vi "Handle Events.vi"(8 "error in (no error)":errorcluster, 11 "TreeControlEventHandler":refnum<class "TreeControlEventHandler.lvclass">) -> ()   [LabVIEW 2019, in "ActorEvents.lvlib" / "TreeControlEventHandler.lvclass"]
uses:
  <vilib>/gpm_packages/@cs/mva-viewable/Source/ActorEvents/EventHandler/TreeControlEventHandler/TreeControlEventHandler.lvclass
  C:/Program Files/National Instruments/LabVIEW 2019/vi.lib/gpm_packages/@cs/mva-viewable/Source/ActorEvents/IEventHandler/IEventHandler.lvclass
  <vilib>/gpm_packages/@cs/mva-viewable/Source/ActorEvents/EventHandler/TreeControlEventHandler/TreeControlEventHandler.lvclass/TreeControlEventHandler.ctl
  <vilib>/gpm_packages/@cs/mva-viewable/Source/ActorEvents/IEventHandler/IEventHandler.lvclass/IEventHandler.ctl
  <vilib>/ActorFramework/Message Enqueuer/Message Enqueuer.lvclass/Message Enqueuer.ctl
  <vilib>/gpm_packages/@cs/mva-viewable/Source/ActorEvents/IEventAggregator Messages/EventDataMessage/EventDataMessage.lvclass/EventDataMessage.ctl
  <vilib>/gpm_packages/@cs/mva-viewable/Source/ActorEvents/IEventAggregator Messages/ControlDragSourceUpdateMsg/ControlDragSourceUpdateMsg.lvclass/ControlDragSourceUpdateMsg.ctl
  <vilib>/gpm_packages/@cs/mva-viewable/Source/ActorEvents/IEventAggregator Messages/ControlDragStartingMsg/ControlDragStartingMsg.lvclass/ControlDragStartingMsg.ctl
  <vilib>/gpm_packages/@cs/mva-viewable/Source/ActorEvents/IEventAggregator Messages/ControlMouseDownMsg/ControlMouseDownMsg.lvclass/ControlMouseDownMsg.ctl
  <vilib>/gpm_packages/@cs/mva-viewable/Source/ActorEvents/IEventAggregator Messages/ControlKeyDownMsg/ControlKeyDownMsg.lvclass/ControlKeyDownMsg.ctl
  <vilib>/event_ctls.llb/lveventtype.ctl
  <vilib>/gpm_packages/@cs/mva-viewable/Source/ActorEvents/IEventAggregator Messages/TreeEditCellMsg/TreeEditCellMsg.lvclass/TreeEditCellMsg.ctl
  <vilib>/gpm_packages/@cs/mva-viewable/Source/ActorEvents/IEventAggregator Messages/EventDataMessage/Read Discarded.vi
  <vilib>/gpm_packages/@cs/mva-viewable/Source/ActorEvents/IEventAggregator Messages/ControlDragSourceUpdateMsg/Accessors/Read Cursor.vi
  <vilib>/gpm_packages/@cs/mva-viewable/Source/ActorEvents/IEventAggregator Messages/ControlDragStartingMsg/Accessors/Read Data.vi
  <vilib>/gpm_packages/@cs/mva-viewable/Source/ActorEvents/IEventAggregator Messages/ControlDragStartingMsg/Accessors/Read Drag Mode.vi
  <vilib>/gpm_packages/@cs/mva-viewable/Source/ActorEvents/IEventAggregator Messages/ControlMouseDownMsg/Accessors/Read Button.vi
  <vilib>/gpm_packages/@cs/mva-viewable/Source/ActorEvents/IEventAggregator Messages/ControlMouseDownMsg/Accessors/Read Mods.vi
  <vilib>/gpm_packages/@cs/mva-viewable/Source/ActorEvents/IEventAggregator Messages/ControlMouseDownMsg/Accessors/Read PlatMods.vi
  <vilib>/gpm_packages/@cs/mva-viewable/Source/ActorEvents/IEventAggregator Messages/ControlKeyDownMsg/Accessors/Read Char.vi
  <vilib>/gpm_packages/@cs/mva-viewable/Source/ActorEvents/IEventAggregator Messages/ControlKeyDownMsg/Accessors/Read VKey.vi
  <vilib>/gpm_packages/@cs/mva-viewable/Source/ActorEvents/IEventAggregator Messages/ControlKeyDownMsg/Accessors/Read Mods.vi
  <vilib>/gpm_packages/@cs/mva-viewable/Source/ActorEvents/IEventAggregator Messages/ControlKeyDownMsg/Accessors/Read PlatMods.vi
  <vilib>/gpm_packages/@cs/mva-viewable/Source/ActorEvents/IEventAggregator Messages/ControlKeyDownMsg/Accessors/Read FocusObj.vi
  <vilib>/gpm_packages/@cs/mva-viewable/Source/ActorEvents/IEventAggregator Messages/TreeEditCellMsg/Accessors/Read String.vi
  <vilib>/gpm_packages/@cs/mva-viewable/Source/ActorEvents/IEventHandler/Accessors/Read Timeout [ms].vi
  <vilib>/gpm_packages/@cs/mva-viewable/Source/ActorEvents/IEventHandler/Accessors/Read Event Filter.vi
  <vilib>/gpm_packages/@cs/mva-viewable/Source/ActorEvents/IEventHandler/Accessors/Read EventAggregator Enqueuer.vi
  <vilib>/gpm_packages/@cs/mva-viewable/Source/ActorEvents/IEventHandler/Accessors/Read Timeout Message.vi
  <vilib>/gpm_packages/@cs/mva-viewable/Source/ActorEvents/IEventHandler/Accessors/Read Timeout Message Priority.vi
  <vilib>/gpm_packages/@cs/mva-viewable/Source/ActorEvents/IEventAggregator Messages/ControlDropMsg/ControlDropMsg.lvclass
  C:/Program Files/National Instruments/LabVIEW 2019/vi.lib/gpm_packages/@cs/mva-viewable/Source/ActorEvents/IEventAggregator Messages/EventDataMessage/EventDataMessage.lvclass
  <vilib>/gpm_packages/@cs/mva-viewable/Source/ActorEvents/IEventAggregator Messages/ControlDragOverMsg/ControlDragOverMsg.lvclass
  <vilib>/gpm_packages/@cs/mva-viewable/Source/ActorEvents/IEventAggregator Messages/ControlDragSourceUpdateMsg/ControlDragSourceUpdateMsg.lvclass
  <vilib>/gpm_packages/@cs/mva-viewable/Source/ActorEvents/IEventAggregator Messages/ControlDragStartingMsg/ControlDragStartingMsg.lvclass
  <vilib>/gpm_packages/@cs/mva-viewable/Source/ActorEvents/IEventAggregator Messages/ControlMouseDownMsg/ControlMouseDownMsg.lvclass
  <vilib>/gpm_packages/@cs/mva-viewable/Source/ActorEvents/IEventAggregator Messages/ControlKeyDownMsg/ControlKeyDownMsg.lvclass
  <vilib>/gpm_packages/@cs/mva-viewable/Source/ActorEvents/IEventAggregator Messages/TreeItemOpenMsg/TreeItemOpenMsg.lvclass
  <vilib>/gpm_packages/@cs/mva-viewable/Source/ActorEvents/IEventAggregator Messages/TreeItemCloseMsg/TreeItemCloseMsg.lvclass
  <vilib>/gpm_packages/@cs/mva-viewable/Source/ActorEvents/IEventAggregator Messages/ShortcutMenuActivationMsg/ShortcutMenuActivationMsg.lvclass
  <vilib>/gpm_packages/@cs/mva-viewable/Source/ActorEvents/IEventAggregator Messages/ShortcutMenuSelectionMsg/ShortcutMenuSelectionMsg.lvclass
  <vilib>/gpm_packages/@cs/mva-viewable/Source/ActorEvents/IEventAggregator Messages/TreeEditCellMsg/TreeEditCellMsg.lvclass
  <vilib>/ActorFramework/Message Priority Queue/Priority Enqueue.vi
  <vilib>/gpm_packages/@cs/mva-viewable/Source/ActorEvents/IEventFilter/IEventFilter.lvclass
  <vilib>/ActorFramework/Message Enqueuer/Message Enqueuer.lvclass
  <vilib>/ActorFramework/Message/Message.lvclass
  <vilib>/gpm_packages/@cs/mva-viewable/Source/ActorEvents/IEventAggregator Messages/ValueChangeMsg/ValueChangeMsg.lvclass
  <vilib>/gpm_packages/@cs/mva-viewable/Source/ActorEvents/IEventAggregator Messages/ControlMouseUpMsg/ControlMouseUpMsg.lvclass
  <vilib>/gpm_packages/@cs/mva-viewable/Source/ActorEvents/IEventAggregator Messages/TreeDoubleClickMsg/TreeDoubleClickMsg.lvclass
  <vilib>/gpm_packages/@cs/mva-viewable/Source/ActorEvents/IEventAggregator Messages/ControlMouseEnterMsg/ControlMouseEnterMsg.lvclass
  <vilib>/gpm_packages/@cs/mva-viewable/Source/ActorEvents/IEventAggregator Messages/ControlMouseLeaveMsg/ControlMouseLeaveMsg.lvclass
  <vilib>/gpm_packages/@cs/mva-viewable/Source/ActorEvents/IEventAggregator Messages/ControlKeyUpMsg/ControlKeyUpMsg.lvclass
  <vilib>/gpm_packages/@cs/mva-viewable/Source/ActorEvents/IEventAggregator Messages/ControlDragEndedMsg/ControlDragEndedMsg.lvclass
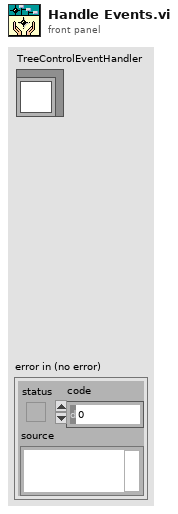
[diagram p1: front panel]
types:
  T1 = typedef "ActorEvents.lvlib/IEventFilter.lvclass/EventFilter Reference.ctl" = refnum<data-value>
  T2 = typedef "Actor Framework.lvlib/Message Enqueuer.lvclass/Message Priority.ctl" = enum16{"Low", "Normal", "High"}
  T3 = typedef "lveventtype.ctl" = enum32{"Null", "Timeout", "Annotation Menu Selection", "Annotation Menu Selection?", "App Instance Close", "App Instance Close?", "Autoscale Range Change", "Bookmark Info Change", "Cell Edit", "Cell Edit?", "Cursor Grab", "Cursor Grab?", "Cursor Menu Selection", "Cursor Menu Selection?", "Cursor Move", "Cursor Release", "Data Change", "Direction Change", "Display State Change", "Drag Ended", "Drag Enter", "Drag Leave", "Drag Over", "Drag Source Update", "Drag Starting", "Drag Starting?", "Drop", "Exec State Change", "Key Down", "Key Down?", "Key Repeat", "Key Repeat?", "Key Up", "Listbox Double Click", "Menu Activation?", "Menu Selection (App)", "Menu Selection? (App)", "Menu Selection (User)", "Mouse Down", "Mouse Down?", "Mouse Enter", "Mouse Leave", "Mouse Move", "Mouse Up", "Mouse Wheel", "NI Security User Change (App)", "Pane Size", "Panel Close", "Panel Close?", "Panel Resize", "Plot Attribute Change", "Scale Range Change", "Shortcut Menu Activation?", "Shortcut Menu Selection (App)", "Shortcut Menu Selection? (App)", "Shortcut Menu Selection (User)", "Tree Double Click", "Tree Drag", "Tree Drag?", "Tree Drop", "Tree Drop?", "Tree Item Close", "Tree Item Close?", "Tree Item Open", "Tree Item Open?", "User Event", "Value Change"}
  T4 = typedef "LVPoint32TypeDef.ctl" = cluster{"Horizontal":i32, "Vertical":i32}
  T5 = cluster{"Shift":bool, "Ctrl":bool, "Alt":bool, "Cmd":bool, "Opt":bool}
  T6 = cluster{"data name":string, "drag data":variant}[]
  T7 = typedef "eventvkey.ctl" = enum16{"ASCII", "Enter", "Return", "Shift", "Ctrl", "Alt", "Cmd", "Opt", "Caps", "NumLock", "Clear", "Break", "Up", "Down", "Left", "Right", "Insert", "Delete", "Home", "End", "PageUp", "PageDown", "Escape", "Help", "Pause", "ScrollLock", "F1", "F2", "F3", "F4", "F5", "F6", "F7", "F8", "F9", "F10", "F11", "F12", "F13", "F14", "F15", "F16", "F17", "F18", "F19", "F20", "F21", "F22", "F23", "F24", "Play", "VolumeUp", "VolumeDown", "Mute", "Two Byte Char"}
  T8 = enum16{"Text", "Background", "Item Symbol", "Open/Close Symbol", "Hierarchy Lines", "Right Border", "Bottom Border", "Bottom Right Corner", "Unknown Part"}
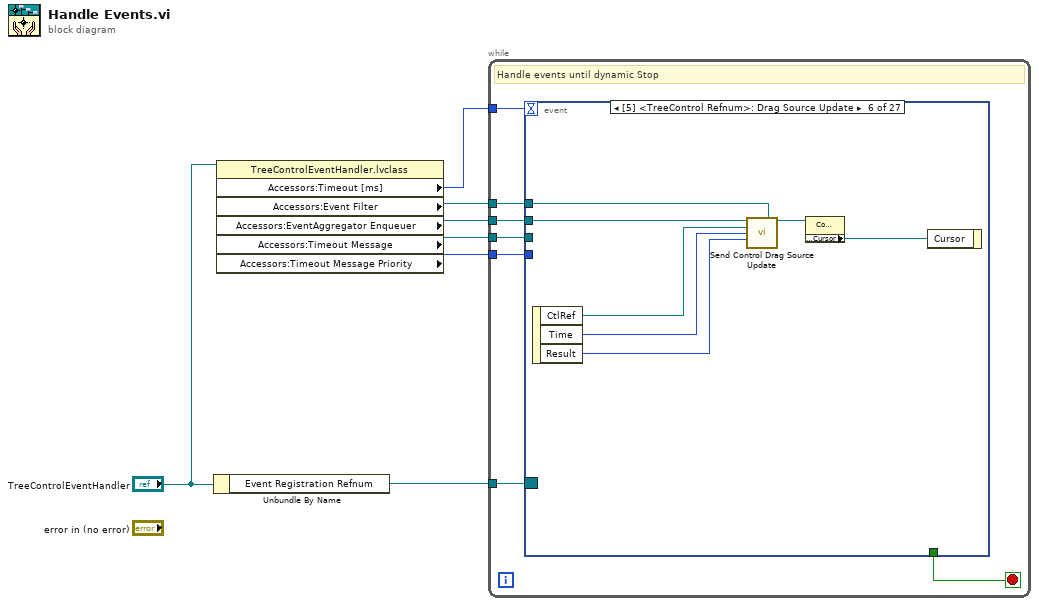
[diagram p0: block diagram]
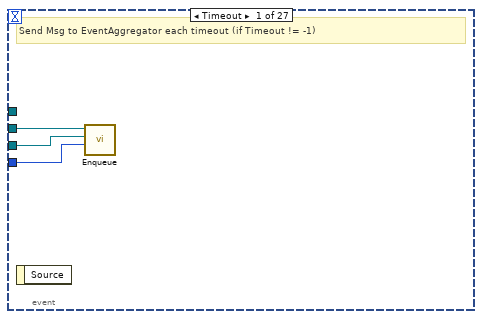
[diagram p2: hidden frame]
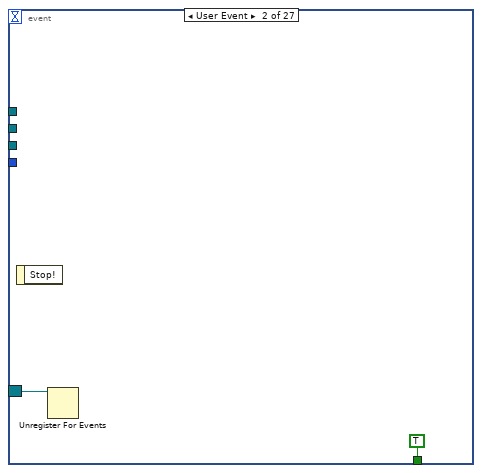
[diagram p3: hidden frame]
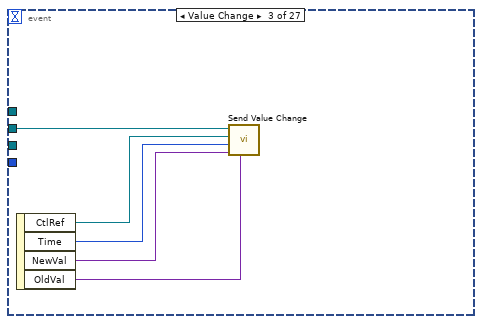
[diagram p4: hidden frame]
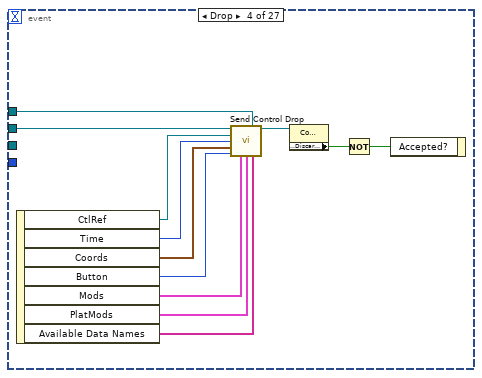
[diagram p5: hidden frame]
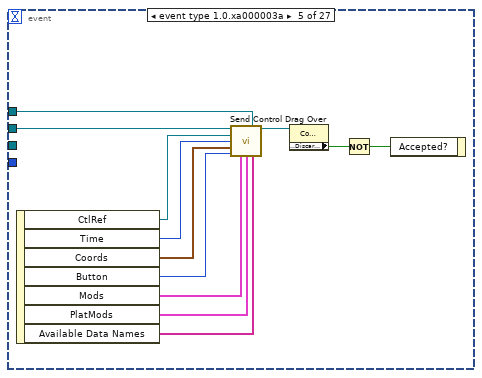
[diagram p6: hidden frame]
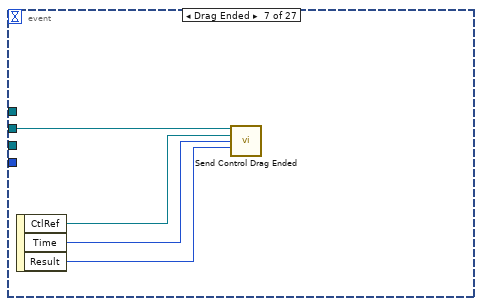
[diagram p7: hidden frame]
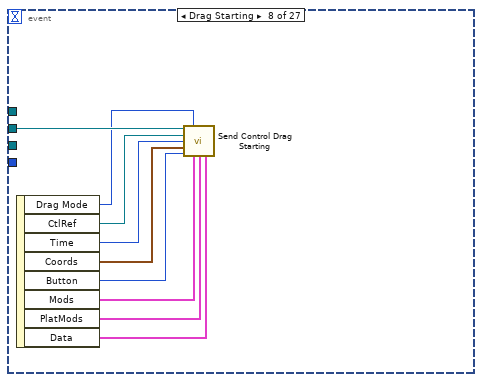
[diagram p8: hidden frame]
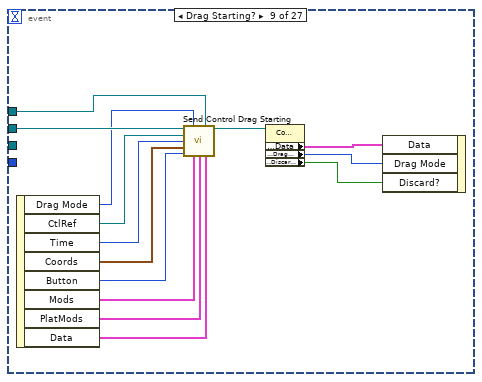
[diagram p9: hidden frame]
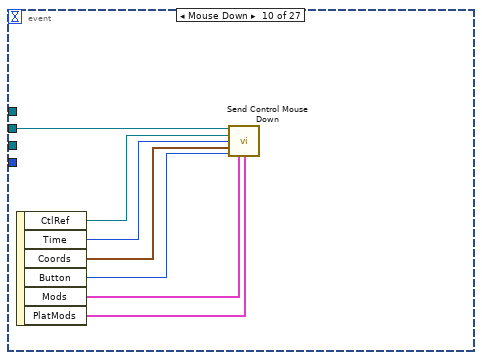
[diagram p10: hidden frame]
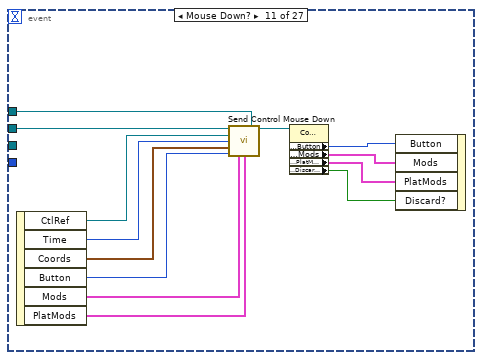
[diagram p11: hidden frame]
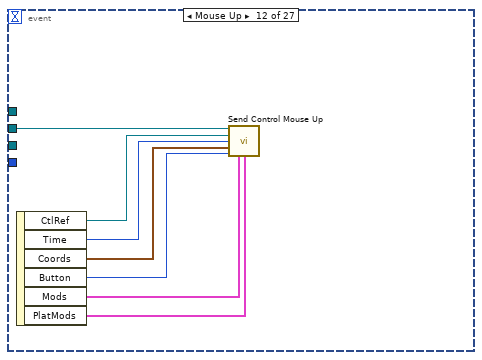
[diagram p12: hidden frame]
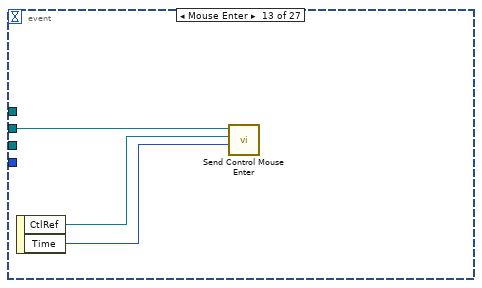
[diagram p13: hidden frame]
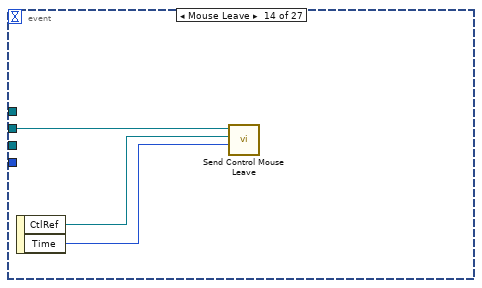
[diagram p14: hidden frame]
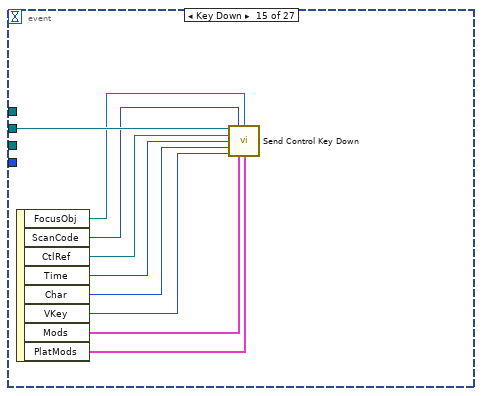
[diagram p15: hidden frame]
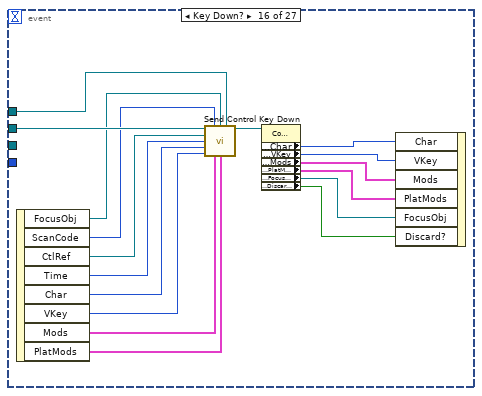
[diagram p16: hidden frame]
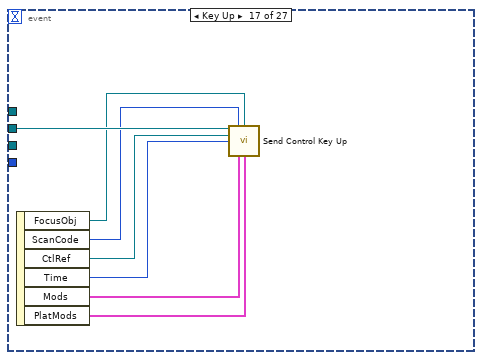
[diagram p17: hidden frame]
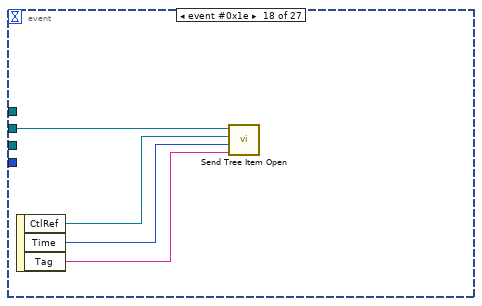
[diagram p18: hidden frame]
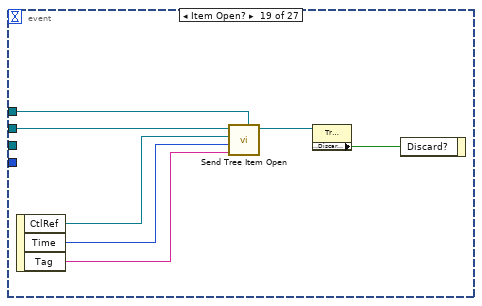
[diagram p19: hidden frame]
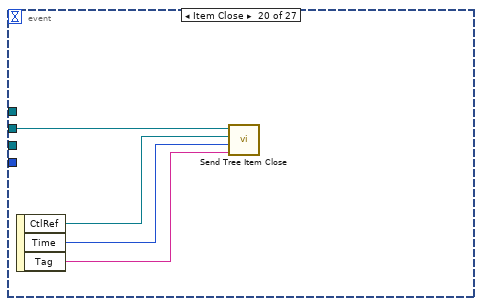
[diagram p20: hidden frame]
diagram:
  n1 = Unbundle By Name("TreeControlEventHandler") -> ("Event Registration Refnum"=w7:refnum<event-registration>)
  n2 = property class="TreeControlEventHandler.lvclass"(reference="TreeControlEventHandler") -> ("Accessors:Timeout [ms]"=w5:i32, "Accessors:Event Filter"=w1:T1, "Accessors:EventAggregator Enqueuer"=w4:refnum<class "Message Enqueuer.lvclass">, "Accessors:Timeout Message"=w3:refnum<class "Message.lvclass">, "Accessors:Timeout Message Priority"=w2:T2)  [unwired: 1 in, 2 out]
  n3 = while {
    tunnel: w7 -> [w14]
    tunnel: w4 -> [w13]
    tunnel: w3 -> [w12]
    tunnel: w5 -> [w11]
    tunnel: w2 -> [w9]
    tunnel: w1 -> [w8]
    stop <- w10 stop-if-true
    # "Handle events until dynamic Stop"
    n4 = event shown="[5] <TreeControl Refnum>: Drag Source Update" {
      selector: w14 -> [_ w19 _ _ _ _ _ _ _ _ _ _ _ _ _ _ _ _ _ _ _ _ _ _ _ _ _]
      dyn-events: _ -> [_ _ _ _ _ _ _ _ _ _ _ _ _ _ _ _ _ _ _ _ _ _ _ _ _ _ _]
      timeout: w11 -> [_ _ _ _ _ _ _ _ _ _ _ _ _ _ _ _ _ _ _ _ _ _ _ _ _ _ _]
      tunnel: [_ TRUE ("Stop!") _ _ _ _ _ _ _ _ _ _ _ _ _ _ _ _ _ _ _ _ _ _ _ _ _] -> w10
      tunnel: w13 -> [w17 _ w24 w36 w48 w55 w59 w68 w82 w89 w102 w109 w112 w115 w124 w141 w148 w152 w159 w163 w170 w179 w188 w198 w209 w215 w225]
      tunnel: w12 -> [w16 _ _ _ _ _ _ _ _ _ _ _ _ _ _ _ _ _ _ _ _ _ _ _ _ _ _]
      tunnel: w9 -> [w15 _ _ _ _ _ _ _ _ _ _ _ _ _ _ _ _ _ _ _ _ _ _ _ _ _ _]
      tunnel: w8 -> [_ _ _ w28 w41 w52 _ _ w73 _ w95 _ _ _ _ w132 _ _ w155 _ w166 _ w182 _ w202 _ w219]
      event Timeout {
        # "Send Msg to EventAggregator each timeout (if Timeout != -1)"
        n5 = event-data() -> ()  [unwired: 1 in, 1 out]
        n6 = call <vilib>:"Enqueue.vi"("Message Priority (Normal)"=w15, "Message"=w16, "Message Enqueuer in"=w17) -> ()  [unwired: 7 in, 2 out]
      }
      event User Event {
        n7 = event-data() -> ()  [unwired: 1 in, 1 out]
        n8 = Unregister For Events(event registration refnum=w19) -> ()  [unwired: 1 in, 1 out]
      }
      event Value Change {
        n9 = event-data() -> ("CtlRef"=w21:refnum<vi>, "Time"=w23:u32, "NewVal"=w22:variant, "OldVal"=w20:variant)  [unwired: 1 in]
        n10 = call <vilib>:"Send Value Change.vi"("Old Value"=w20, "New Value"=w22, "Time"=w23, "Ctl Refnum"=w21, "Message Enqueuer in"=w24) -> ()  [unwired: 6 in, 1 out]
      }
      event Drop {
        n11 = event-data() -> ("CtlRef"=w35:refnum<vi>, "Time"=w34:u32, "Coords"=w33:T4, "Button"=w32:u16, "Mods"=w31:cluster{"Double Click":bool, "Menu Key":bool}, "PlatMods"=w30:T5, "Available Data Names"=w29:string[])  [unwired: 1 in]
        n12 = call <vilib>:"Send Control Drop.vi"("Message Enqueuer in"=w36, "EventFilter Reference"=w28, "CtlRef"=w35, "Time"=w34, "Coords"=w33, "Button"=w32, "Mods"=w31, "PlatMods"=w30, "Available Data Names"=w29) -> ("Filtered EventDataMessage"=w27:refnum<class "ControlDropMsg.lvclass">)  [unwired: 5 in, 1 out]
        n13 = property class="ControlDropMsg.lvclass"(reference=w27) -> ("Accessors:Discarded?"=w26:bool)  [unwired: 1 in, 2 out]
        n14 = Not(x=w26) -> (.not. x?=w25:bool)
        n15 = event-data("Accepted?"=w25) -> ()  [unwired: 1 in, 1 out]
      }
      event event type 1.0.xa000003a {
        n16 = event-data() -> ("CtlRef"=w47:refnum<vi>, "Time"=w46:u32, "Coords"=w45:T4, "Button"=w44:u16, "Mods"=w43:cluster{"Double Click":bool, "Menu Key":bool}, "PlatMods"=w42:T5, "Available Data Names"=w37:string[])  [unwired: 1 in]
        n17 = call <vilib>:"Send Control Drag Over.vi"("Message Enqueuer in"=w48, "EventFilter Reference"=w41, "CtlRef"=w47, "Time"=w46, "Coords"=w45, "Button"=w44, "Mods"=w43, "PlatMods"=w42, "Available Data Names"=w37) -> ("Filtered EventDataMessage"=w40:refnum<class "ControlDragOverMsg.lvclass">)  [unwired: 5 in, 1 out]
        n18 = property class="ControlDragOverMsg.lvclass"(reference=w40) -> ("Accessors:Discarded?"=w39:bool)  [unwired: 1 in, 2 out]
        n19 = Not(x=w39) -> (.not. x?=w38:bool)
        n20 = event-data("Accepted?"=w38) -> ()  [unwired: 1 in, 1 out]
      }
      event Drag Source Update {
        n21 = event-data() -> ("CtlRef"=w54:refnum<vi>, "Time"=w53:u32, "Result"=w49:enum16{"Drop Cancel", "Drop Move", "Drop Copy"})  [unwired: 1 in]
        n22 = call <vilib>:"Send Control Drag Source Update.vi"("Message Enqueuer in"=w55, "EventFilter Reference"=w52, "CtlRef"=w54, "Time"=w53, "Result"=w49) -> ("Filtered EventDataMessage"=w51:refnum<class "ControlDragSourceUpdateMsg.lvclass">)  [unwired: 9 in, 1 out]
        n23 = property class="ControlDragSourceUpdateMsg.lvcl"(reference=w51) -> ("Accessors:Cursor"=w50:refnum<k1>)  [unwired: 1 in, 2 out]
        n24 = event-data("Cursor"=w50) -> ()  [unwired: 1 in, 1 out]
      }
      event Drag Ended {
        n25 = event-data() -> ("CtlRef"=w58:refnum<vi>, "Time"=w57:u32, "Result"=w56:enum16{"Drop Cancel", "Drop Move", "Drop Copy"})  [unwired: 1 in]
        n26 = call <vilib>:"Send Control Drag Ended.vi"("Message Enqueuer in"=w59, "CtlRef"=w58, "Time"=w57, "Result"=w56) -> ()  [unwired: 10 in, 2 out]
      }
      event Drag Starting {
        n27 = event-data() -> ("Drag Mode"=w67:enum32{"copy or move", "copy only", "move only"}, "CtlRef"=w66:refnum<vi>, "Time"=w65:u32, "Coords"=w64:T4, "Button"=w63:u16, "Mods"=w62:cluster{"Double Click":bool, "Menu Key":bool}, "PlatMods"=w61:T5, "Data"=w60:T6)  [unwired: 1 in]
        n28 = call <vilib>:"Send Control Drag Starting.vi"("Message Enqueuer in"=w68, "Drag Mode"=w67, "CtlRef"=w66, "Time"=w65, "Coords"=w64, "Button"=w63, "Mods"=w62, "PlatMods"=w61, "Data"=w60) -> ()  [unwired: 5 in, 2 out]
      }
      event Drag Starting? {
        n29 = event-data() -> ("Drag Mode"=w81:enum32{"copy or move", "copy only", "move only"}, "CtlRef"=w80:refnum<vi>, "Time"=w79:u32, "Coords"=w78:T4, "Button"=w77:u16, "Mods"=w76:cluster{"Double Click":bool, "Menu Key":bool}, "PlatMods"=w75:T5, "Data"=w74:T6)  [unwired: 1 in]
        n30 = call <vilib>:"Send Control Drag Starting.vi"("Message Enqueuer in"=w82, "Drag Mode"=w81, "EventFilter Reference"=w73, "CtlRef"=w80, "Time"=w79, "Coords"=w78, "Button"=w77, "Mods"=w76, "PlatMods"=w75, "Data"=w74) -> ("Filtered EventDataMessage"=w72:refnum<class "ControlDragStartingMsg.lvclass">)  [unwired: 4 in, 1 out]
        n31 = property class="ControlDragStartingMsg.lvclass"(reference=w72) -> ("Accessors:Data"=w71:T6, "Accessors:Drag Mode"=w70:enum32{"copy or move", "copy only", "move only"}, "Accessors:Discarded?"=w69:bool)  [unwired: 1 in, 2 out]
        n32 = event-data("Data"=w71, "Drag Mode"=w70, "Discard?"=w69) -> ()  [unwired: 1 in, 1 out]
      }
      event Mouse Down {
        n33 = event-data() -> ("CtlRef"=w88:refnum<vi>, "Time"=w87:u32, "Coords"=w86:T4, "Button"=w85:u16, "Mods"=w84:cluster{"Double Click":bool, "Menu Key":bool}, "PlatMods"=w83:T5)  [unwired: 1 in]
        n34 = call <vilib>:"Send Control Mouse Down.vi"("Message Enqueuer in"=w89, "Ctl Refnum"=w88, "Time"=w87, "Coords"=w86, "Button"=w85, "Mods"=w84, "PlatMods"=w83) -> ()  [unwired: 7 in, 2 out]
      }
      event Mouse Down? {
        n35 = event-data() -> ("CtlRef"=w101:refnum<vi>, "Time"=w100:u32, "Coords"=w99:T4, "Button"=w98:u16, "Mods"=w97:cluster{"Double Click":bool, "Menu Key":bool}, "PlatMods"=w96:T5)  [unwired: 1 in]
        n36 = call <vilib>:"Send Control Mouse Down.vi"("Message Enqueuer in"=w102, "EventFilter Reference"=w95, "Ctl Refnum"=w101, "Time"=w100, "Coords"=w99, "Button"=w98, "Mods"=w97, "PlatMods"=w96) -> ("Filtered EventDataMessage"=w94:refnum<class "ControlMouseDownMsg.lvclass">)  [unwired: 6 in, 1 out]
        n37 = property class="ControlMouseDownMsg.lvclass"(reference=w94) -> ("Accessors:Button"=w93:u16, "Accessors:Mods"=w92:cluster{"Double Click":bool, "Menu Key":bool}, "Accessors:PlatMods"=w91:T5, "Accessors:Discarded?"=w90:bool)  [unwired: 1 in, 2 out]
        n38 = event-data("Button"=w93, "Mods"=w92, "PlatMods"=w91, "Discard?"=w90) -> ()  [unwired: 1 in, 1 out]
      }
      event Mouse Up {
        n39 = event-data() -> ("CtlRef"=w108:refnum<vi>, "Time"=w107:u32, "Coords"=w106:T4, "Button"=w105:u16, "Mods"=w104:cluster{"Double Click":bool, "Menu Key":bool}, "PlatMods"=w103:T5)  [unwired: 1 in]
        n40 = call <vilib>:"Send Control Mouse Up.vi"("Message Enqueuer in"=w109, "Ctl Refnum"=w108, "Time"=w107, "Coords"=w106, "Button"=w105, "Mods"=w104, "PlatMods"=w103) -> ()  [unwired: 8 in, 1 out]
      }
      event Mouse Enter {
        n41 = event-data() -> ("CtlRef"=w111:refnum<vi>, "Time"=w110:u32)  [unwired: 1 in]
        n42 = call <vilib>:"Send Control Mouse Enter.vi"("Time"=w110, "Ctl Refnum"=w111, "Message Enqueuer in"=w112) -> ()  [unwired: 8 in, 1 out]
      }
      event Mouse Leave {
        n43 = event-data() -> ("CtlRef"=w114:refnum<vi>, "Time"=w113:u32)  [unwired: 1 in]
        n44 = call <vilib>:"Send Control Mouse Leave.vi"("Time"=w113, "Ctl Refnum"=w114, "Message Enqueuer in"=w115) -> ()  [unwired: 8 in, 1 out]
      }
      event Key Down {
        n45 = event-data() -> ("FocusObj"=w123:refnum<vi>, "ScanCode"=w122:i16, "CtlRef"=w121:refnum<vi>, "Time"=w120:u32, "Char"=w119:i16, "VKey"=w118:T7, "Mods"=w117:cluster{"Num Pad":bool, "Menu Key":bool}, "PlatMods"=w116:T5)  [unwired: 1 in]
        n46 = call <vilib>:"Send Control Key Down.vi"("Message Enqueuer in"=w124, "ScanCode"=w122, "FocusObj"=w123, "CtlRef"=w121, "Time"=w120, "Char"=w119, "VKey"=w118, "Mods"=w117, "PlatMods"=w116) -> ()  [unwired: 5 in, 2 out]
      }
      event Key Down? {
        n47 = event-data() -> ("FocusObj"=w140:refnum<vi>, "ScanCode"=w139:i16, "CtlRef"=w138:refnum<vi>, "Time"=w137:u32, "Char"=w136:i16, "VKey"=w135:T7, "Mods"=w134:cluster{"Num Pad":bool, "Menu Key":bool}, "PlatMods"=w133:T5)  [unwired: 1 in]
        n48 = call <vilib>:"Send Control Key Down.vi"("Message Enqueuer in"=w141, "ScanCode"=w139, "FocusObj"=w140, "EventFilter Reference"=w132, "CtlRef"=w138, "Time"=w137, "Char"=w136, "VKey"=w135, "Mods"=w134, "PlatMods"=w133) -> ("Filtered EventDataMessage"=w131:refnum<class "ControlKeyDownMsg.lvclass">)  [unwired: 4 in, 1 out]
        n49 = property class="ControlKeyDownMsg.lvclass"(reference=w131) -> ("Accessors:Char"=w130:i16, "Accessors:VKey"=w129:T7, "Accessors:Mods"=w128:cluster{"Double Click":bool, "Menu Key":bool}, "Accessors:PlatMods"=w127:T5, "Accessors:FocusObj"=w126:refnum<vi>, "Accessors:Discarded?"=w125:bool)  [unwired: 1 in, 2 out]
        n50 = event-data("Char"=w130, "VKey"=w129, "Mods"=w128, "PlatMods"=w127, "FocusObj"=w126, "Discard?"=w125) -> ()  [unwired: 1 in, 1 out]
      }
      event Key Up {
        n51 = event-data() -> ("FocusObj"=w147:refnum<vi>, "ScanCode"=w146:i16, "CtlRef"=w145:refnum<vi>, "Time"=w144:u32, "Mods"=w143:cluster{"Num Pad":bool, "Menu Key":bool}, "PlatMods"=w142:T5)  [unwired: 1 in]
        n52 = call <vilib>:"Send Control Key Up.vi"("Message Enqueuer in"=w148, "ScanCode"=w146, "FocusObj"=w147, "Ctl Refnum"=w145, "Time"=w144, "Mods"=w143, "PlatMods"=w142) -> ()  [unwired: 8 in, 1 out]
      }
      event event #0x1e {
        n53 = event-data() -> ("CtlRef"=w151:refnum<vi>, "Time"=w150:u32, "Tag"=w149:string)  [unwired: 1 in]
        n54 = call <vilib>:"Send Tree Item Open.vi"("Item Tag"=w149, "Time"=w150, "CtlRef"=w151, "Message Enqueuer in"=w152) -> ()  [unwired: 6 in, 2 out]
      }
      event Item Open? {
        n55 = event-data() -> ("CtlRef"=w158:refnum<vi>, "Time"=w157:u32, "Tag"=w156:string)  [unwired: 1 in]
        n56 = call <vilib>:"Send Tree Item Open.vi"("EventFilter Reference"=w155, "Item Tag"=w156, "Time"=w157, "CtlRef"=w158, "Message Enqueuer in"=w159) -> ("Filtered EventDataMessage"=w154:refnum<class "TreeItemOpenMsg.lvclass">)  [unwired: 5 in, 1 out]
        n57 = property class="TreeItemOpenMsg.lvclass"(reference=w154) -> ("Accessors:Discarded?"=w153:bool)  [unwired: 1 in, 2 out]
        n58 = event-data("Discard?"=w153) -> ()  [unwired: 1 in, 1 out]
      }
      event Item Close {
        n59 = event-data() -> ("CtlRef"=w162:refnum<vi>, "Time"=w161:u32, "Tag"=w160:string)  [unwired: 1 in]
        n60 = call <vilib>:"Send Tree Item Close.vi"("Item Tag"=w160, "Time"=w161, "CtlRef"=w162, "Message Enqueuer in"=w163) -> ()  [unwired: 6 in, 2 out]
      }
      event event type 1.0.x80000011 {
        n61 = event-data() -> ("CtlRef"=w169:refnum<vi>, "Time"=w168:u32, "Tag"=w167:string)  [unwired: 1 in]
        n62 = call <vilib>:"Send Tree Item Close.vi"("EventFilter Reference"=w166, "Item Tag"=w167, "Time"=w168, "CtlRef"=w169, "Message Enqueuer in"=w170) -> ("Filtered EventDataMessage"=w165:refnum<class "TreeItemCloseMsg.lvclass">)  [unwired: 5 in, 1 out]
        n63 = property class="TreeItemCloseMsg.lvclass"(reference=w165) -> ("Accessors:Discarded?"=w164:bool)  [unwired: 1 in, 2 out]
        n64 = event-data("Discard?"=w164) -> ()  [unwired: 1 in, 1 out]
      }
      event Double Click {
        n65 = event-data() -> ("CellPart"=w171:T8, "Tag"=w172:string, "CtlRef"=w178:refnum<vi>, "Time"=w177:u32, "Coords"=w176:T4, "Button"=w175:u16, "Mods"=w174:cluster{"Double Click":bool, "Menu Key":bool}, "PlatMods"=w173:T5)  [unwired: 1 in]
        n66 = call <vilib>:"Send Tree Double Click.vi"("Message Enqueuer in"=w179, "Tag"=w172, "CellPart"=w171, "Tree Refnum"=w178, "Time"=w177, "Coords"=w176, "Button"=w175, "Mods"=w174, "PlatMods"=w173) -> ()  [unwired: 6 in, 1 out]
      }
      event Shortcut Menu Activation? {
        n67 = event-data() -> ("CtlRef"=w183:refnum<vi>, "Time"=w187:u32, "MenuRef"=w184:refnum<k9>, "Coords"=w186:T4, "SubObj"=w185:refnum<vi>)  [unwired: 1 in]
        n68 = call <vilib>:"Send Shortcut Menu Activation.vi"("Message Enqueuer in"=w188, "EventFilter Reference"=w182, "CtlRef"=w183, "Time"=w187, "MenuRef"=w184, "Coords"=w186, "SubObj"=w185) -> ("Filtered EventDataMessage"=w181:refnum<class "ShortcutMenuActivationMsg.lvclass">)  [unwired: 7 in, 1 out]
        n69 = property class="ShortcutMenuActivationMsg.lvcla"(reference=w181) -> ("Accessors:Discarded?"=w180:bool)  [unwired: 1 in, 2 out]
        n70 = event-data("Discard?"=w180) -> ()  [unwired: 1 in, 1 out]
      }
      event Shortcut Menu Selection (User); Shortcut Menu Selection (App) {
        n71 = event-data() -> ("Type"=w191:T3, "CtlRef"=w197:refnum<vi>, "Time"=w196:u32, "ItemTag"=w195:string, "ItemPath"=w194:string, "Coords"=w193:T4, "SubObj"=w192:refnum<vi>)  [unwired: 1 in]
        n72 = Equal?(x=lveventtype."Shortcut Menu Selection (App)", y=w191) -> (x = y?=w190:bool)
        n73 = call <vilib>:"Send Shortcut Menu Selection.vi"("Message Enqueuer in"=w198, "App Item?"=w190, "CtlRef"=w197, "Time"=w196, "Item Tag"=w195, "Item Path"=w194, "Coords"=w193, "SubObj"=w192) -> ()  [unwired: 6 in, 2 out]
      }
      event Shortcut Menu Selection? (App) {
        w200 = TRUE  # App Item?
        n74 = event-data() -> ("CtlRef"=w208:refnum<vi>, "Time"=w207:u32, "ItemTag"=w206:string, "ItemPath"=w205:string, "Coords"=w204:T4, "SubObj"=w203:refnum<vi>)  [unwired: 1 in]
        n75 = call <vilib>:"Send Shortcut Menu Selection.vi"("Message Enqueuer in"=w209, "App Item?"=w200, "EventFilter Reference"=w202, "CtlRef"=w208, "Time"=w207, "Item Tag"=w206, "Item Path"=w205, "Coords"=w204, "SubObj"=w203) -> ("Filtered EventDataMessage"=w201:refnum<class "ShortcutMenuSelectionMsg.lvclass">)  [unwired: 5 in, 1 out]
        n76 = property class="ShortcutMenuSelectionMsg.lvclas"(reference=w201) -> ("Accessors:Discarded?"=w199:bool)  [unwired: 1 in, 2 out]
        n77 = event-data("Discard?"=w199) -> ()  [unwired: 1 in, 1 out]
      }
      event Edit Cell {
        n78 = event-data() -> ("CtlRef"=w214:refnum<vi>, "Time"=w213:u32, "String"=w212:string, "Tag"=w211:string, "Col"=w210:i32)  [unwired: 1 in]
        n79 = call <vilib>:"Send Tree Edit Cell.vi"("Col"=w210, "Tag"=w211, "String"=w212, "Time"=w213, "CtlRef"=w214, "Message Enqueuer in"=w215) -> ()  [unwired: 4 in, 2 out]
      }
      event Edit Cell? {
        n80 = event-data() -> ("CtlRef"=w224:refnum<vi>, "Time"=w223:u32, "String"=w222:string, "Tag"=w221:string, "Col"=w220:i32)  [unwired: 1 in]
        n81 = call <vilib>:"Send Tree Edit Cell.vi"("Col"=w220, "EventFilter Reference"=w219, "Tag"=w221, "String"=w222, "Time"=w223, "CtlRef"=w224, "Message Enqueuer in"=w225) -> ("Filtered EventDataMessage"=w218:refnum<class "TreeEditCellMsg.lvclass">)  [unwired: 3 in, 1 out]
        n82 = property class="TreeEditCellMsg.lvclass"(reference=w218) -> ("Accessors:String"=w217:string, "Accessors:Discarded?"=w216:bool)  [unwired: 1 in, 2 out]
        n83 = event-data("String"=w217, "Discard?"=w216) -> ()  [unwired: 1 in, 1 out]
      }
    }
  }
